vi "set current.vi"(8 "error in (no error)":errorcluster, 10 "Current [A]":dbl, 11 "generic-power-supply in":refnum<class "generic-power-supply.lvclass">) -> (0 "error out":errorcluster, 3 "generic-power-supply out":refnum<class "generic-power-supply.lvclass">)   [LabVIEW 2025, in "Power Supply.lvlib" / "generic-power-supply.lvclass"]
uses:
  generic-power-supply.lvclass
  generic-power-supply.lvclass/generic-power-supply.ctl
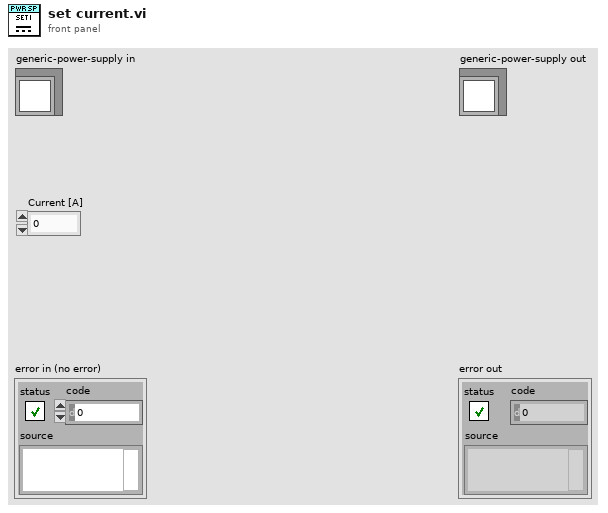
[diagram p1: front panel]
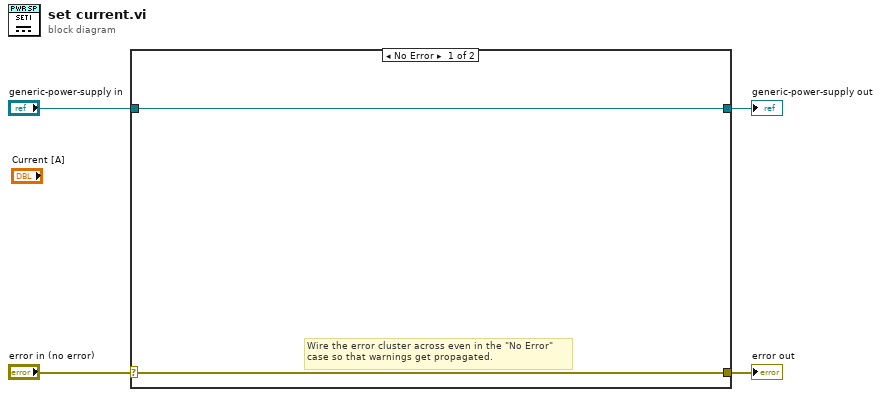
[diagram p0: block diagram]
diagram:
  n1 = case shown="No Error" "error in (no error)" {
    selector: "error in (no error)" -> [w5 w8]
    tunnel: [w5 w8] -> w3
    tunnel: [w6 w7] -> w1
    tunnel: "generic-power-supply in" -> [w6 w7]
    frame No Error {
      # "Wire the error cluster across even in the \"No Error\"\ncase so that warnings get propagated."
    }
    frame Error {
    }
  }
  "error out" <- w3
  "generic-power-supply out" <- w1
